vi "Motor_Plus_Impedance_controller_sunday.vi"() -> ()   [LabVIEW 2016]
uses:
  <vilib>/Platform/TimedLoop/XDataNode/timing_clust.ctl
  <vilib>/Platform/TimedLoop/XDataNode/nitl_modes.ctl
  <vilib>/Platform/TimedLoop/XDataNode/wakeup.ctl
  <vilib>/Platform/TimedLoop/XDataNode/loadnilvce.vi
  <vilib>/Motion/Express/_s/nimc.ax.power.power.axis.vi
  <vilib>/Motion/Express/_s/nimc.fb.read.readExecutionData.axis.vi
  <vilib>/Motion/Express/_s/nimc.fb.straightLineMove.startStraightLineMove.axis.modeVelocity.0.vi
  <vilib>/Motion/Express/_s/nimc.fb.stopMove.stop.axis.modeDecelerate.vi
  <vilib>/Motion/Express/_s/nimc.fb.resetPosition.resetPosition.axis.vi
  <vilib>/Motion/Express/_s/nimc.ex.power.power.axis.vi
  <vilib>/platform/TimedLoop/XDataNode/XDataNode.xnode
  <vilib>/Motion/BlockNode/FB.NIMotion.xnode
  <vilib>/Platform/TimedLoop/XDataNode/XDNodeRunTimeDep.lvlib
panel:
  out "Adjusted Motor Velocity":dbl format="%.3f"
  out "Adjusted Velocity":dbl(knob) scale=0.0..3.0
  in  "Reset Position":bool
  in  "Position":dbl=0.25 format="%#_13g"
  in  "Speed":dbl=0.25 format="%#_13g"
  out "Torque":dbl(knob) scale=-5.0..5.0
  out "Position":dbl(knob) scale=0.0..1.0
  out "Velocity":dbl(knob) scale=0.0..5.0
  out "Load Cell":dbl(knob) scale=0.0..10.0
  in  "desired motor\nposition":dbl
  in  "Move to Position?":bool
  out "Load cell, V":dbl format="%.3f"
  out "motor torque, Nm":dbl format="%.3f"
  out "motor velocity, rev/s":dbl format="%.3f"
  out "motor position, rev":dbl format="%.3f"
  in  "STOP VI":bool
  in  "Enable Axis \nControl":bool
  in  "Enable Motor \nDrive":bool
  in  "EMERGENCY MOTOR STOP":bool
  # "Raw Data from System"
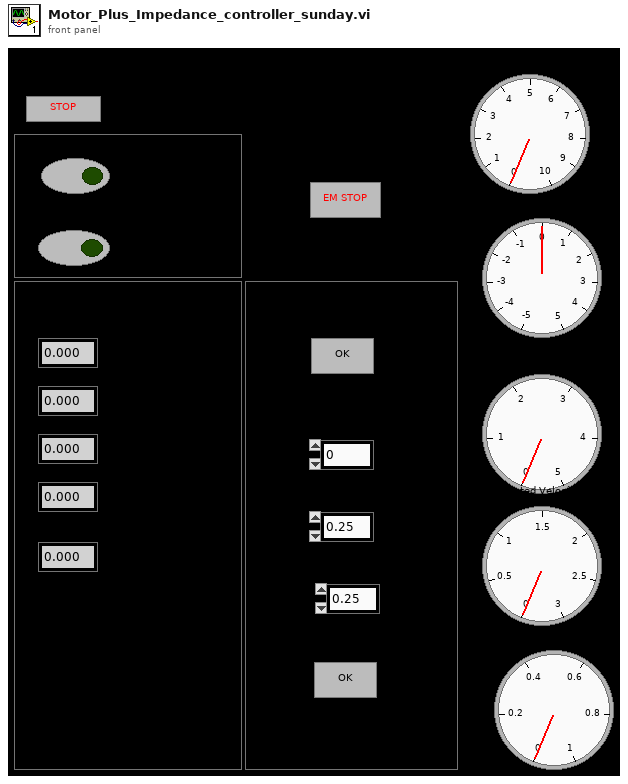
[diagram p1: front panel]
types:
  T1 = typedef "XDNodeRunTimeDep.lvlib/timing_clust.ctl" = cluster{"Expected End [f-1]":u64, "Actual End [f-1]":u64, "Finished Late? [f-1]":bool, "Expected End [i-1]":u64, "Actual End [i-1]":u64, "Finished Late? [i-1]":bool, "Expected Start [i]":u64, "Actual Start [i]":u64, "Expected Start [f]":u64, "Actual Start [f]":u64, "Source Name":string, "Structure Name":string, "Period":i64, "Deadline":i64, "Offset":i64, "Start":i64, "Priority":i32, "Timeout":i32, "Mode":T2, "Wakeup Reason":T3, "Error":errorcluster, "Source Type":string, "Secondary Source Type":string, "Global End Time":u64, "Global Start Time":u64, "Frame Duration":u64, "Iteration Duration":u64, "Assigned CPU":i32, "I/O Scan Engine Mode":u32}
  T2 = typedef "XDNodeRunTimeDep.lvlib/nitl_modes.ctl" = enum32{"No Change", "Process missed periods, maintain original phase", "Discard missed periods, maintain original phase", "Process missed periods, ignore original phase", "Discard missed periods, ignore original phase"}
  T3 = typedef "XDNodeRunTimeDep.lvlib/wakeup.ctl" = enum32{"Normal", "Aborted", "Asynchronous wakeup", "Timing source error", "Timed loop error", "Timeout"}
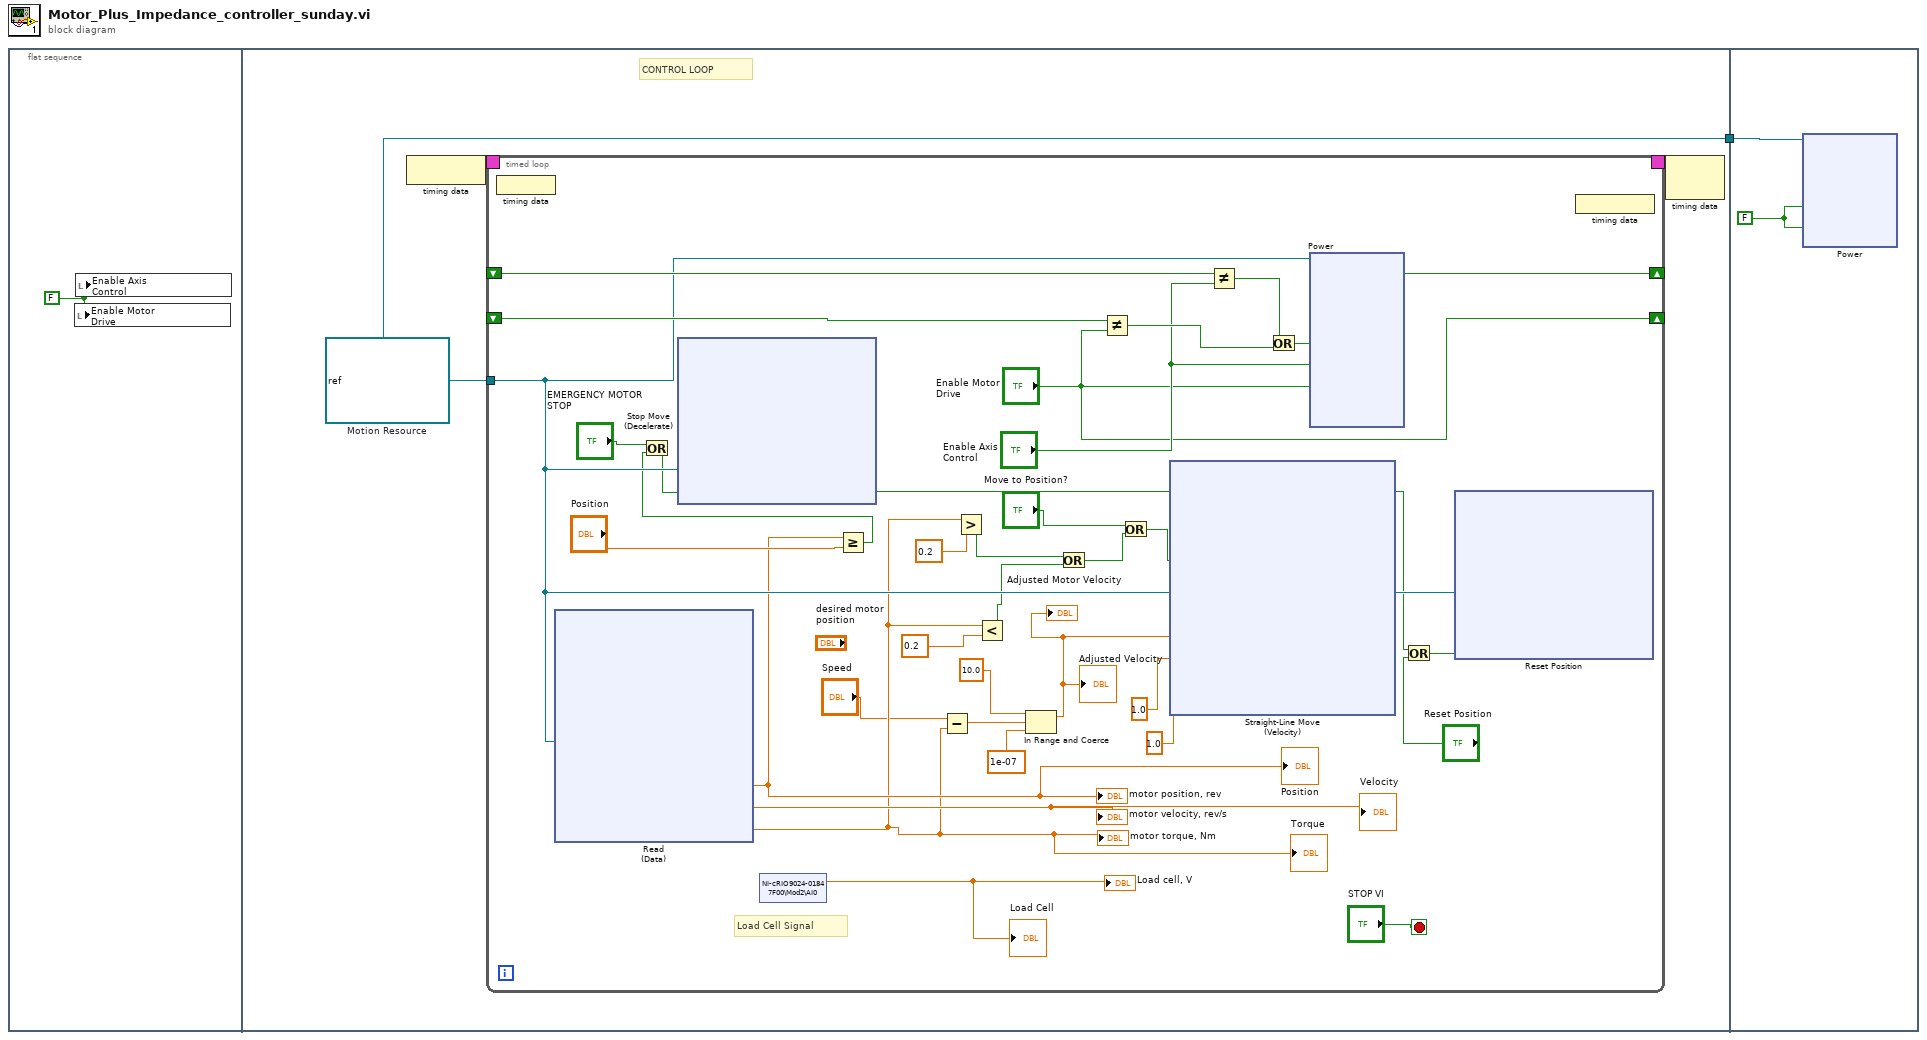
[diagram p0: block diagram]
diagram:
  n1 = flat-sequence {
    tunnel: [w5] -> w1
    tunnel: w1 -> [w118]
    frame #0 {
      w2 = FALSE
      n2 = local write "Enable Motor \nDrive"(w2) -> ()
      n3 = local write "Enable Axis \nControl"(w2) -> ()
    }
    frame #1 {
      w5 = refnum<k21> "nism://NI-cRIO9024-01847F00/Axis 1"  # Motion Resource
      # "CONTROL LOOP"
      n4 = node-c288() -> (w4:T1)
      n5 = timed-loop {
        tunnel: w5 -> [w31]
        timing: w4 -> [_]
        timing-out: [_] -> w3
        shift-right: ["Enable Axis \nControl"] -> _
        shift-left: _ -> [w39]
        shift-right: ["Enable Motor \nDrive"] -> _
        shift-left: _ -> [w38]
        stop <- "STOP VI" stop-if-true
        # "Load Cell Signal"
        n6 = node-c288() -> ()  [unwired: 1 in]
        n7 = xnode "Read\n(Data)"("resource"=w31) -> ("position"=w22:dbl, "torque"=w10:dbl, "velocity"=→"motor velocity, rev/s" →"Velocity":dbl)  [unwired: 1 in, 3 out]
        "motor position, rev" <- w22
        "motor torque, Nm" <- w10
        "Position" <- w22
        "Torque" <- w10
        n8 = shared-variable "NI-cRIO9024-01847F00\\Mod2\\AI0"() -> (→"Load cell, V" →"Load Cell":dbl)  [unwired: 1 in, 1 out]
        n9 = Greater Or Equal?(x=w22, y="Position") -> (x >= y?=w13:bool)
        n10 = Or(x="EMERGENCY MOTOR STOP", y=w13) -> (x .or. y?=w15:bool)
        n11 = xnode "Stop Move\n(Decelerate)"("resource"=w31, "execute"=w15) -> ("done"=w23:bool)  [unwired: 1 in, 2 out]
        n12 = Subtract(x="Speed", y=w10) -> (x-y=w11:dbl)
        n13 = Greater?(x=w10, y=0.2) -> (0:w19:bool)
        n14 = Less?(x=w10, y=0.2) -> (x < y?=w17:bool)
        n15 = In Range and Coerce(upper limit=10.0, x=w11, lower limit=1e-07) -> (coerced(x)=w21:dbl)  [unwired: 1 out]
        "Adjusted Velocity" <- w21
        "Adjusted Motor Velocity" <- w21
        n16 = Or(x=w19, y=w17) -> (x .or. y?=w7:bool)
        n17 = Not Equal?(x=w38, y="Enable Motor \nDrive") -> (x != y?=w36:bool)
        n18 = Or(x="Move to Position?", y=w7) -> (x .or. y?=w8:bool)
        n19 = xnode "Straight-Line Move\n(Velocity)"("resource"=w31, "execute"=w8, "velocity"=w21, "acceleration"=1.0, "deceleration"=1.0) -> ("resource out"=w27:refnum<k21>)  [unwired: 1 in, 2 out]
        n20 = Not Equal?(x=w39, y="Enable Axis \nControl") -> (x != y?=w37:bool)
        n21 = Or(x=w37, y=w36) -> (x .or. y?=w35:bool)
        n22 = xnode ("Power")("execute"=w35, "enable axis"="Enable Axis \nControl", "enable drive"="Enable Motor \nDrive", "resource"=w31) -> ()  [unwired: 1 in, 6 out]
        n23 = Or(x=w23, y="Reset Position") -> (x .or. y?=w26:bool)
        n24 = xnode "Reset Position"("resource"=w27, "execute"=w26) -> ()  [unwired: 2 in, 3 out]
        n25 = node-c288() -> ()  [unwired: 1 out]
      }
      n26 = node-c288(w3) -> ()  [unwired: 1 out]
    }
    frame #2 {
      w119 = FALSE
      n27 = xnode ("Power")("enable axis"=w119, "enable drive"=w119, "resource"=w118) -> ()  [unwired: 1 in, 2 out]
    }
  }
